vi "MMI_BCM_StrDismantle.vi"(1 "LogEvent":refnum<vi>, 2 "VCI_CAN_OBJ_R":T1) -> (0 "BCM_CmdCluster":T2 {"天窗开度" scale=0.0..100.0; "语音命令天窗开关" items=["默认", "停止"]; "右后侧车窗开度" scale=0.0..100.0; "左后侧车窗开度" scale=0.0..100.0; "副驾驶侧车窗开度" scale=0.0..100.0; "驾驶侧车窗开度" scale=0.0..100.0; "伴我回家时间" items=["无", "30s", "60s", "90s"]; "门解锁设置应答" items=["无应答", "应答驾驶门解锁", "应答所有门解锁"]; "天窗翘起控制" items=["无", "倾斜翘起", "倾斜关闭"]; "车窗防夹报警" items=["无", "禁止", "启用"]; "日间行车灯" items=["无", "禁止", "启用"]; "智能弯道灯" items=["无", "禁止", "启用"]; "后视镜自动折叠" items=["无", "禁止", "启用"]; "下雨关窗模式" items=["无", "关", "开"]; "设防提示类型" items=["无", "亮灯并鸣笛", "亮灯", "鸣笛"]})   [LabVIEW 2013]
uses:
  Log.ctl
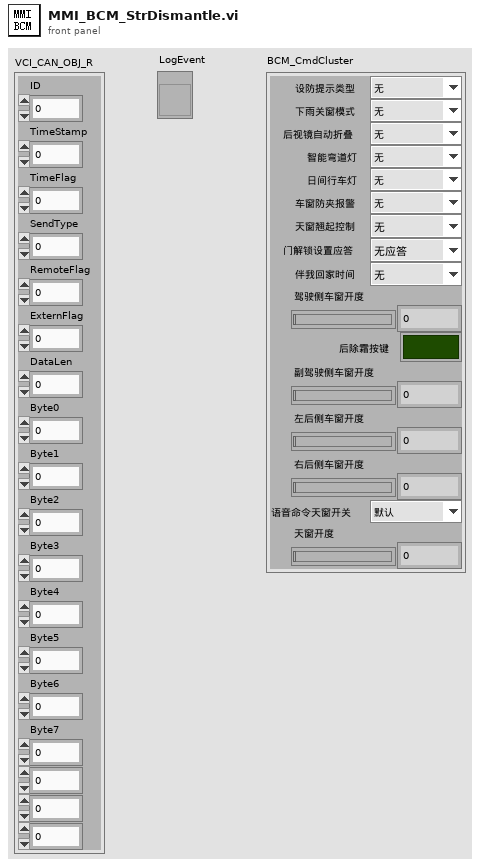
[diagram p1: front panel]
types:
  T1 = cluster{"ID":u32, "TimeStamp":u32, "TimeFlag":u8, "SendType":u8, "RemoteFlag":u8, "ExternFlag":u8, "DataLen":u8, "Byte0":u8, "Byte1":u8, "Byte2":u8, "Byte3":u8, "Byte4":u8, "Byte5":u8, "Byte6":u8, "Byte7":u8, u8, u8, u8}
  T2 = cluster{"设防提示类型":u16, "下雨关窗模式":u16, "后视镜自动折叠":u16, "智能弯道灯":u16, "日间行车灯":u16, "车窗防夹报警":u16, "天窗翘起控制":u16, "门解锁设置应答":u16, "伴我回家时间":u16, "驾驶侧车窗开度":u8, "后除霜按键":bool, "副驾驶侧车窗开度":u8, "左后侧车窗开度":u8, "右后侧车窗开度":u8, "语音命令天窗开关":u16, "天窗开度":u8}
  T3 = typedef "Log.ctl" = cluster{"Event":string, "Value":variant}
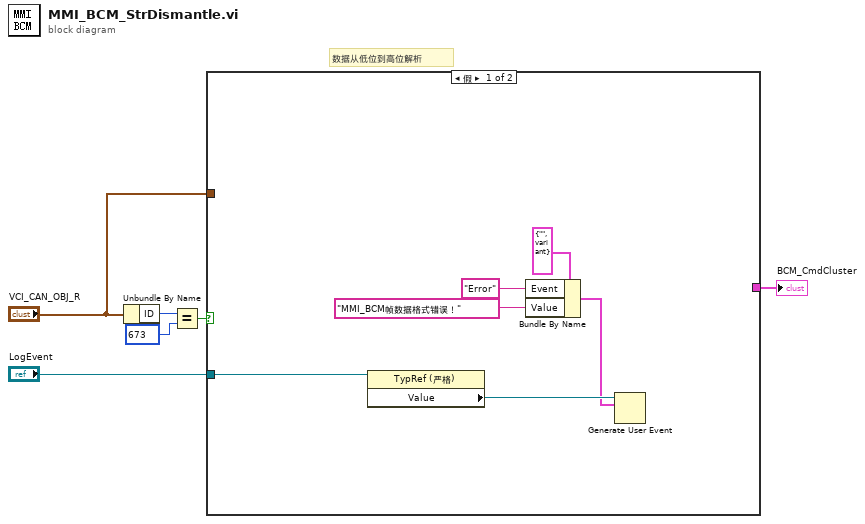
[diagram p0: block diagram]
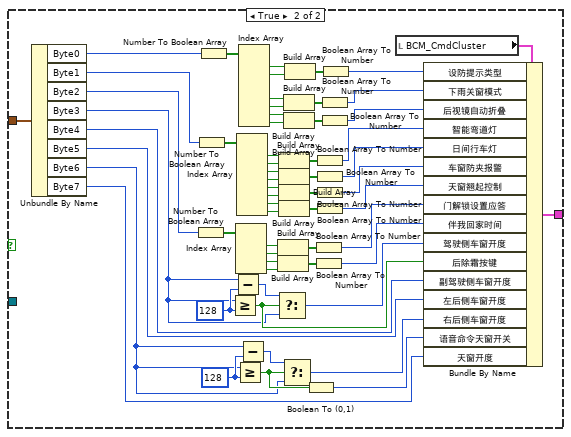
[diagram p2: hidden frame]
diagram:
  # "数据从低位到高位解析"
  n1 = Unbundle By Name("VCI_CAN_OBJ_R") -> ("ID"=w5:u32)
  n2 = Equal?(x=w5, y=u16 673) -> (x = y?=w3:bool)
  n3 = case shown="假" w3 {
    tunnel: [_ w69] -> w6
    tunnel: "VCI_CAN_OBJ_R" -> [_ w21]
    tunnel: "LogEvent" -> [w8 _]
    frame False {
      n4 = property class="TypRef (严格)"(reference=w8) -> ("Value"=w12:refnum<user-event>)  [unwired: 1 in, 2 out]
      n5 = Bundle By Name(cluster=T3 {"Event"="", "Value"=variant} ("Log"), "Event"="Error", "Value"="MMI_BCM帧数据格式错误！" ("消息")) -> (w9:T3)
      n6 = Generate User Event(user event=w12, event data cluster=w9) -> ()  [unwired: 2 in, 2 out]
    }
    frame True {
      w26 = 128
      w29 = 128
      n7 = Unbundle By Name(w21) -> ("Byte0"=w20:u8, "Byte1"=w19:u8, "Byte2"=w18:u8, "Byte3"=w17:u8, "Byte4"=w16:u8, "Byte5"=w15:u8, "Byte6"=w14:u8, "Byte7"=w13:u8)
      n8 = Number To Boolean Array(number=w18) -> (Boolean array=w39:bool[])
      n9 = Number To Boolean Array(number=w19) -> (Boolean array=w56:bool[])
      n10 = Number To Boolean Array(number=w20) -> (Boolean array=w71:bool[])
      n11 = Greater Or Equal?(x=w17, y=w29) -> (x >= y?=w28:bool)
      n12 = Subtract(x=w17, y=w29) -> (x-y=w30:i32)
      n13 = Greater Or Equal?(x=w14, y=w26) -> (x >= y?=w23:bool)
      n14 = Index Array(array=w39) -> (element #1=w36:bool, element #2=w35:bool, element #3=w34:bool, element #4=w33:bool)  [unwired: 4 in]
      n15 = Index Array(array=w56) -> (element #1=w52:bool, element #2=w51:bool, element #3=w49:bool, element #4=w48:bool, element #5=w47:bool, element #6=w46:bool, element #7=w45:bool, element #8=w44:bool)  [unwired: 8 in]
      n16 = Subtract(x=w14, y=w26) -> (x-y=w25:i32)
      n17 = Index Array(array=w71) -> (element #1=w68:bool, element #2=w67:bool, element #5=w64:bool, element #6=w63:bool, element #7=w59:bool, element #8=w58:bool)  [unwired: 8 in, 2 out]
      n18 = Select(t=w30, s=w28, f=w17) -> (s? t:f=w27:i32)
      n19 = Build Array(w36, w35) -> (w37:bool[])
      n20 = Build Array(w34, w33) -> (w38:bool[])
      n21 = Build Array(w52, w51) -> (w53:bool[])
      n22 = Build Array(w49, w48) -> (w50:bool[])
      n23 = Build Array(w47, w46) -> (w54:bool[])
      n24 = Build Array(w45, w44) -> (w55:bool[])
      n25 = Select(t=w25, s=w23, f=w14) -> (s? t:f=w24:i32)
      n26 = Build Array(w64, w63) -> (w62:bool[])
      n27 = Build Array(w59, w58) -> (w60:bool[])
      n28 = Build Array(w68, w67) -> (w66:bool[])
      n29 = Boolean To (0,1)(Boolean=w23) -> (0, 1=w22:i16)
      n30 = Boolean Array To Number(Boolean array=w37) -> (number=w32:u32)
      n31 = Boolean Array To Number(Boolean array=w38) -> (number=w31:u32)
      n32 = Boolean Array To Number(Boolean array=w53) -> (number=w43:u32)
      n33 = Boolean Array To Number(Boolean array=w50) -> (number=w42:u32)
      n34 = Boolean Array To Number(Boolean array=w54) -> (number=w41:u32)
      n35 = Boolean Array To Number(Boolean array=w55) -> (number=w40:u32)
      n36 = Boolean Array To Number(Boolean array=w62) -> (number=w61:u32)
      n37 = Boolean Array To Number(Boolean array=w60) -> (number=w57:u32)
      n38 = Boolean Array To Number(Boolean array=w66) -> (number=w65:u32)
      n39 = local read "BCM_CmdCluster"() -> (w70:T2)
      n40 = Bundle By Name(cluster=w70, "设防提示类型"=w65, "下雨关窗模式"=w61, "后视镜自动折叠"=w57, "智能弯道灯"=w43, "日间行车灯"=w42, "车窗防夹报警"=w41, "天窗翘起控制"=w40, "门解锁设置应答"=w32, "伴我回家时间"=w31, "驾驶侧车窗开度"=w27, "后除霜按键"=w28, "副驾驶侧车窗开度"=w16, "左后侧车窗开度"=w15, "右后侧车窗开度"=w24, "语音命令天窗开关"=w22, "天窗开度"=w13) -> (w69:T2)
    }
  }
  "BCM_CmdCluster" <- w6
